vi "Time Filter Data (unix ns).vi"(4 "End":dbl, 6 "Start":dbl, 10 "Group Data":T2) -> (2 "Data":T1[](array[typedef]))   [LabVIEW 2020, in "VolatusHistorian.lvlib" / "Historian Module.lvclass"]
uses:
  Historian Module.lvclass
  Group Data.ctl
  Channel Data.ctl
  Channel History (unix ns).ctl
  lv-vecto/Vecto/Double to Relative ns (Array).vi
  Historian Module.lvclass/Historian Module.ctl
  VolatusHistorian.lvlib
  lv-vecto/Vecto/Vecto.lvlib
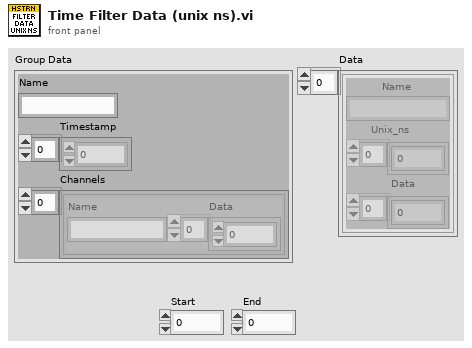
[diagram p1: front panel]
types:
  T1 = typedef "VolatusHistorian.lvlib/Channel History (unix ns).ctl" = cluster{"Name":string, "Unix_ns":i64[], "Data":dbl[]}
  T2 = typedef "VolatusHistorian.lvlib/Group Data.ctl" = cluster{"Name":string, "Timestamp":dbl[], "Channels":T3[]}
  T3 = typedef "VolatusHistorian.lvlib/Channel Data.ctl" = cluster{"Name":string, "Data":dbl[]}
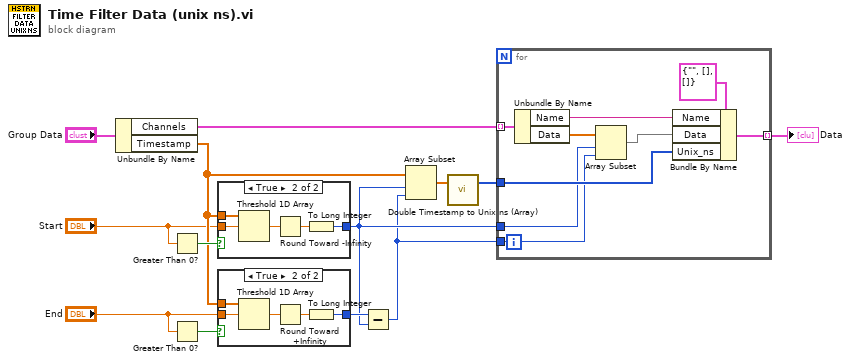
[diagram p0: block diagram]
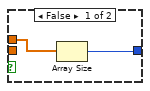
[diagram p2: hidden frame]
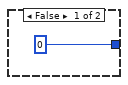
[diagram p3: hidden frame]
diagram:
  n1 = Unbundle By Name("Group Data") -> ("Channels"=w9:T3[], "Timestamp"=w10:dbl[])
  n2 = Greater Than 0?(x="Start") -> (x > 0?=w13:bool)
  n3 = Greater Than 0?(x="End") -> (x > 0?=w12:bool)
  n4 = case shown="True" w13 {
    tunnel: w10 -> [_ w17]
    tunnel: "Start" -> [_ w19]
    tunnel: [0 w16] -> w6
    frame False {
    }
    frame True {
      n5 = Threshold 1D Array(2:w19, 3:w17) -> (0:w18:dbl)  [unwired: 1 in]
      n6 = Round Toward -Infinity(1:w18) -> (0:w15:dbl)
      n7 = To Long Integer(number=w15) -> (32bit integer=w16:i32)
    }
  }
  n8 = case shown="True" w12 {
    tunnel: w10 -> [w21 w24]
    tunnel: "End" -> [_ w26]
    tunnel: [w20 w23] -> w11
    frame False {
      n9 = Array Size(array=w21) -> (size(s)=w20:i32)
    }
    frame True {
      n10 = Threshold 1D Array(2:w26, 3:w24) -> (0:w25:dbl)  [unwired: 1 in]
      n11 = Round Toward +Infinity(x=w25) -> (ceil(x): smallest int >= x=w22:dbl)
      n12 = To Long Integer(number=w22) -> (32bit integer=w23:i32)
    }
  }
  n13 = Subtract(x=w11, y=w6) -> (x-y=w5:i32)
  n14 = Array Subset(array=w10, index=w6, length=w5) -> (w8:dbl[])
  n15 = call "Double Timestamp to Unix ns (Array).vi"("Timestamp"=w8) -> ("unix ns"=w7:i64[])  [unwired: 2 in]
  n16 = for {
    tunnel: w9 -> [w33] mode=indexing
    tunnel: w7 -> [w34]
    tunnel: w6 -> [w30]
    tunnel: w5 -> [w28]
    tunnel: [w27] -> w4 mode=indexing
    n17 = Unbundle By Name(w33) -> ("Name"=w32:string, "Data"=w31:dbl[])
    n18 = Array Subset(array=w31, index=w30, length=w28) -> (w29:dbl[])
    n19 = Bundle By Name(cluster=T1 {"Name"="", "Unix_ns"=[], "Data"=[]} ("Channel History"), "Name"=w32, "Data"=w29, "Unix_ns"=w34) -> (w27:T1)
  }
  "Data" <- w4
